vi "Result_Test.vi"(8 "error in (no error)":errorcluster caption="entrée d'erreur (pas d'erreur)", 11 "Get_Voltage en entrée":refnum<class "Get_Key_DB_AIS.lvclass">) -> (0 "error out":errorcluster caption="sortie d'erreur", 3 "Get_Voltage en sortie":refnum<class "Get_Key_DB_AIS.lvclass">)   [LabVIEW 2020, in "Library Test.lvlib" / "Get_Key_DB_AIS.lvclass"]
uses:
  Get_Key_DB_AIS.lvclass
  C:/Users/ngarcin/OneDrive - Altyor/Standard TB/Class/Test/Test (Default)/Test (Default).lvclass
  Find_SN_In_Database/Find_SN_In_Database.lvclass
  Get_Key_DB_AIS.lvclass/Get_Key_DB_AIS.ctl
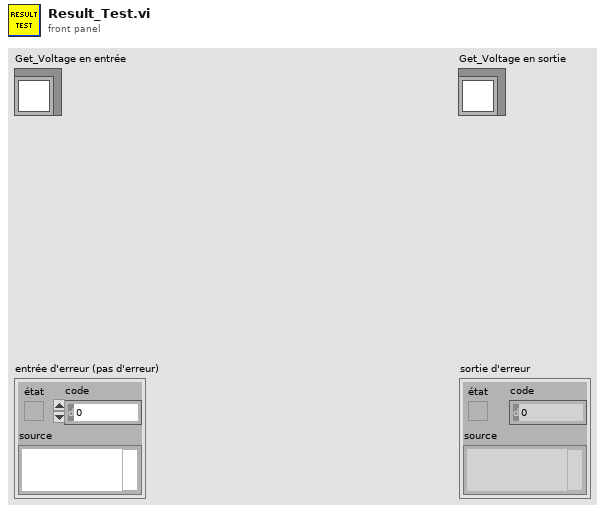
[diagram p1: front panel]
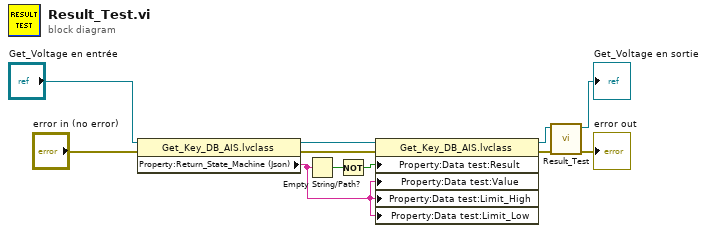
[diagram p0: block diagram]
diagram:
  n1 = property class="Get_Key_DB_AIS.lvclass"(reference="Get_Voltage en entrée", error in="error in (no error)") -> (reference out=w9:refnum<class "Get_Key_DB_AIS.lvclass">, error out=w5:errorcluster, "Property:Return_State_Machine (Json)"=w6:string)
  n2 = Empty String/Path?(string/path=w6) -> (empty?=w4:bool)
  n3 = Not(x=w4) -> (.not. x?=w3:bool)
  n4 = property class="Get_Key_DB_AIS.lvclass"(reference=w9, error in=w5, "Property:Data test:Result"=w3, "Property:Data test:Value"=w6, "Property:Data test:Limit_High"=w6, "Property:Data test:Limit_Low"=w6) -> (reference out=w7:refnum<class "Get_Key_DB_AIS.lvclass">, error out=w8:errorcluster)
  n5 = call-parent "Result_Test.vi"("error in (no error)"=w8, "Generate_SN en entrée"=w7) -> ("error out"=→"error out":errorcluster, "Generate_SN en sortie"=→"Get_Voltage en sortie":refnum<class "Get_Key_DB_AIS.lvclass">)  [unwired: 8 in]
